vi "Lift_State_Machine.vi"() -> ()   [LabVIEW 2016]
doc: "The state machine for the Lift System.\nDrives the lift forward, then upward, then back, then down to its origin."
uses:
  <vilib>/myRIO/Instrument Drivers/Onboard IO/DIO/typedefs/DIO Reference.ctl
  <vilib>/myRIO/Common/Instrument Driver Framework/Utilities/typedefs/myRIO Generic Hardware Reference.ctl
  <vilib>/myRIO/Common/Instrument Driver Framework/Utilities/typedefs/Hardware Version Enum.ctl
  <vilib>/myRIO/Common/Instrument Driver Framework/Utilities/typedefs/myRIO v1.0 Reference.ctl
  <vilib>/myRIO/Common/Instrument Driver Framework/Utilities/typedefs/Generic FPGA Reference.ctl
  <vilib>/myRIO/Common/Instrument Driver Framework/myRIO v1.0/DIO/typedefs/DIO Channels List.ctl
  <vilib>/myRIO/Common/Instrument Driver Framework/myRIO v1.0/DIO/typedefs/DIO Channels Enum.ctl
  <vilib>/userdefined/High Color/nirio_resource_hc.ctl
  <vilib>/myRIO/Common/Instrument Driver Framework/Utilities/vis/Is FPGA Ref Available.vi
  <vilib>/myRIO/Common/Instrument Driver Framework/roboRIO v1.0/DIO/vis/roboRIO v1.0 Open DIO.vi
  <vilib>/myRIO/Instrument Drivers/Onboard IO/DIO/vis/Write.vi
  <vilib>/myRIO/Instrument Drivers/Onboard IO/DIO/vis/Read.vi
  <vilib>/myRIO/Common/Instrument Driver Framework/Utilities/vis/Validate Channels.vi
  <vilib>/myRIO/Common/Instrument Driver Framework/roboRIO v1.0/DIO/vis/roboRIO v1.0 Reserve DIO.vi
  <vilib>/myRIO/Common/Instrument Driver Framework/roboRIO v1.0/DIO/vis/roboRIO v1.0 Build MUX Configuration DIO.vi
  <vilib>/myRIO/Common/Instrument Driver Framework/roboRIO v1.0/Resource Manager/vis/roboRIO v1.0 Reserve Channel List.vi
  <vilib>/myRIO/Common/Instrument Driver Framework/roboRIO v1.0/Resource Manager/vis/roboRIO v1.0 Create Configuration List.vi
  <vilib>/myRIO/Common/Instrument Driver Framework/roboRIO v1.0/Resource Manager/vis/roboRIO v1.0 Reserve Channel.vi
  <vilib>/myRIO/Common/Instrument Driver Framework/roboRIO v1.0/Resource Manager/vis/roboRIO v1.0 Unreserve Channel.vi
  <vilib>/myRIO/Common/Instrument Driver Framework/roboRIO v1.0/Resource Manager/vis/roboRIO v1.0 Build Mutex Name.vi
  GlobalVI.vi
  <vilib>/Utility/VariantDataType/GetNumericInfo.vi
  <vilib>/Utility/error.llb/Error Cluster From Error Code.vi
  <vilib>/myRIO/Common/Instrument Driver Framework/roboRIO v1.0/roboRIO v1.0 Open.vi
  <vilib>/myRIO/Common/Instrument Driver Framework/Utilities/vis/IO Manager.vi
  <vilib>/myRIO/Common/Instrument Driver Framework/Utilities/vis/Configuration Manager.vi
  <vilib>/myRIO/Common/Instrument Driver Framework/roboRIO v1.0/Resource Manager/vis/roboRIO v1.0 Configure IO.vi
  <vilib>/myRIO/Common/Instrument Driver Framework/myRIO v1.0/myRIO v1.0 Close.vi
  <vilib>/myRIO/Common/Instrument Driver Framework/roboRIO v1.0/DIO/vis/roboRIO v1.0 Write DIO.vi
  <vilib>/myRIO/Common/Instrument Driver Framework/roboRIO v1.0/DIO/vis/roboRIO v1.0 Read DIO.vi
  <vilib>/myRIO/Express VI/Onboard IO/DO/DO Express VI.xnode
  <vilib>/myRIO/Instrument Drivers/Onboard IO/DIO/vis/myRIO DIO Open.xnode
  <vilib>/myRIO/Express VI/Onboard Devices/LED/LED Express VI.xnode
  <vilib>/myRIO/Express VI/Onboard IO/DI/DI Express VI.xnode
  <vilib>/myRIO/Instrument Drivers/Onboard IO/DIO/DIO.lvlib
panel:
  out "timeoutError":bool
  out "timeoutCounter":u32
  out "timerCount":u32
  out "liftState":i32
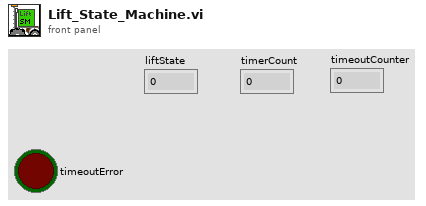
[diagram p1: front panel]
types:
  T1 = typedef "DIO.lvlib/DIO Reference.ctl" = cluster{"myRIO Reference":T2, "DIO Channels List":T6}
  T2 = typedef "myRIO Generic Hardware Reference.ctl" = cluster{"myRIO Model":T3, "myRIO Hardware Reference":T4}
  T3 = typedef "Hardware Version Enum.ctl" = enum16{"Unknown", "myRIO-1900", "myRIO-1950", "roboRIO", "NI ELVIS RIO CM"}
  T4 = typedef "myRIO v1.0 Reference.ctl" = cluster{"Generic FPGA Reference":T5, "Allow multiple opens":bool}
  T5 = typedef "Generic FPGA Reference.ctl" = refnum<k20>
  T6 = typedef "DIO Channels List.ctl" = T7[]
  T7 = typedef "DIO Channels Enum.ctl" = enum16{"Not Connected", "C/DIO0", "C/DIO1", "C/DIO2", "C/DIO3", "C/DIO4", "C/DIO5", "C/DIO6", "C/DIO7", "A/DIO0", "A/DIO1", "A/DIO2", "A/DIO3", "A/DIO4", "A/DIO5", "A/DIO6", "A/DIO7", "A/DIO8", "A/DIO9", "A/DIO10", "A/DIO11", "A/DIO12", "A/DIO13", "A/DIO14", "A/DIO15", "B/DIO0", "B/DIO1", "B/DIO2", "B/DIO3", "B/DIO4", "B/DIO5", "B/DIO6", "B/DIO7", "B/DIO8", "B/DIO9", "B/DIO10", "B/DIO11", "B/DIO12", "B/DIO13", "B/DIO14", "B/DIO15", "LED0", "LED1", "LED2", "LED3", "Button0", "DIO/DIO0", "DIO/DIO1", "DIO/DIO2", "DIO/DIO3", "DIO/DIO4", "DIO/DIO5", "DIO/DIO6", "DIO/DIO7", "DIO/DIO8", "DIO/DIO9", "SPI/CS0", "SPI/CS1", "SPI/CS2", "SPI/CS3", "LED RADIO (Green)", "LED RADIO (Red)", "LED COMM (Green)", "LED COMM (Red)", "LED MODE (Green)", "LED MODE (Red)"}
  T8 = typedef "nirio_resource_hc.ctl" = tag
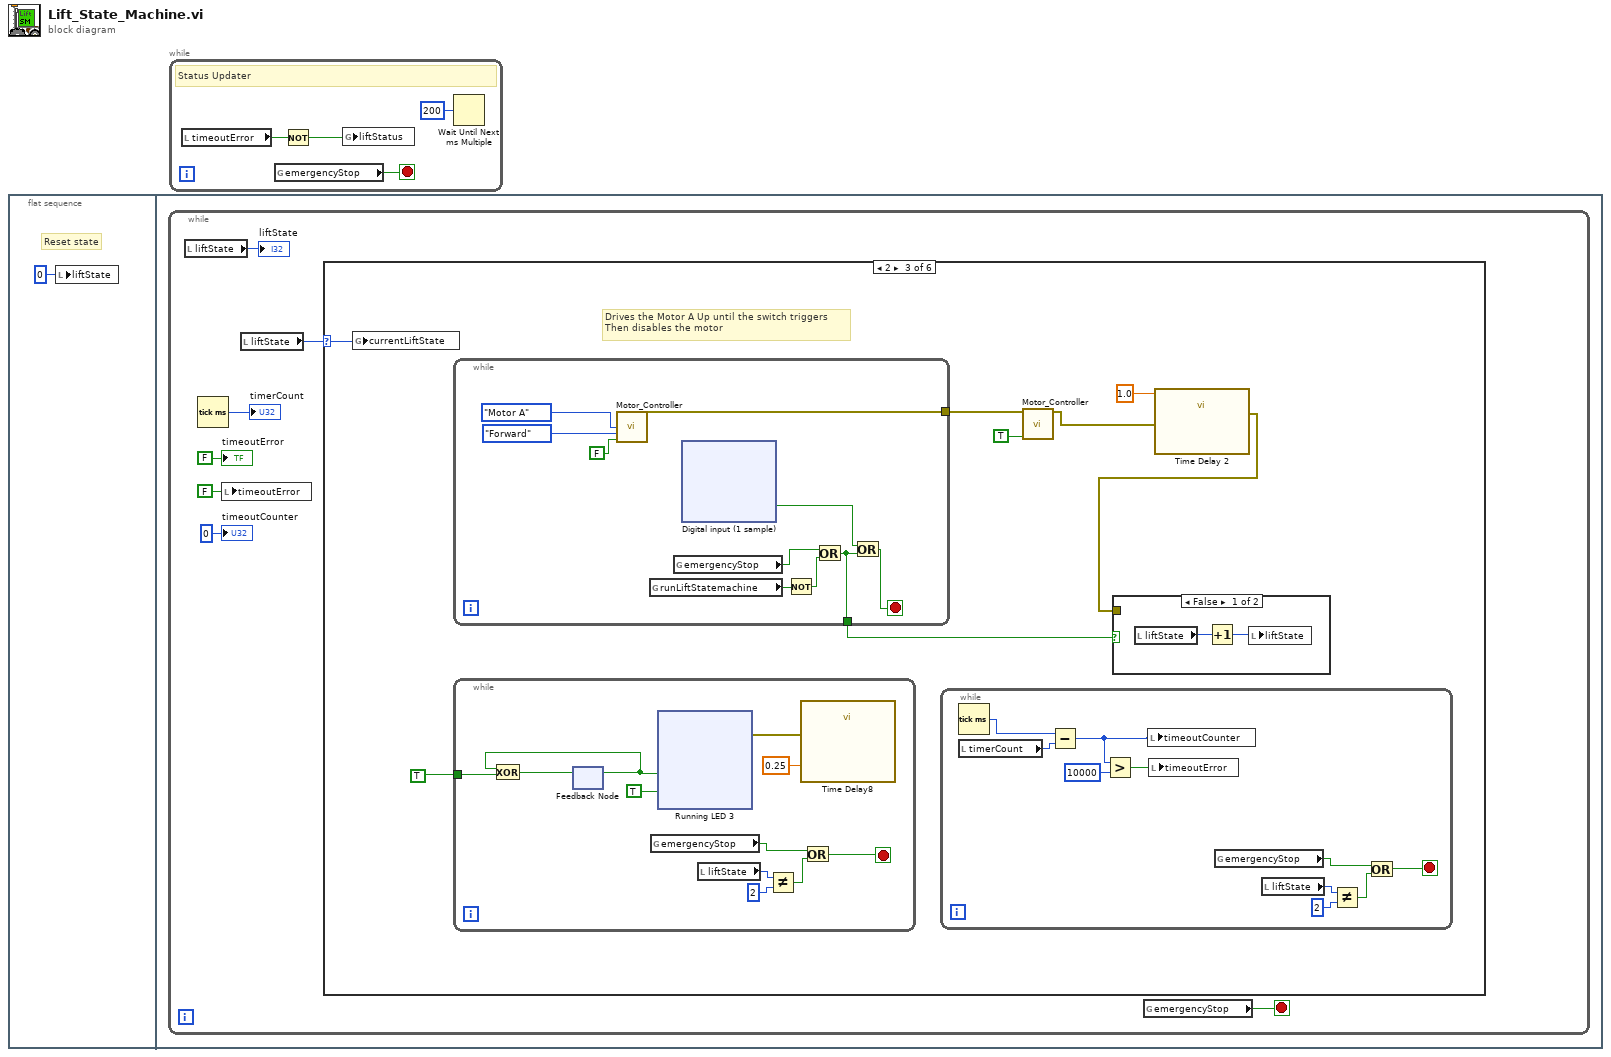
[diagram p0: block diagram]
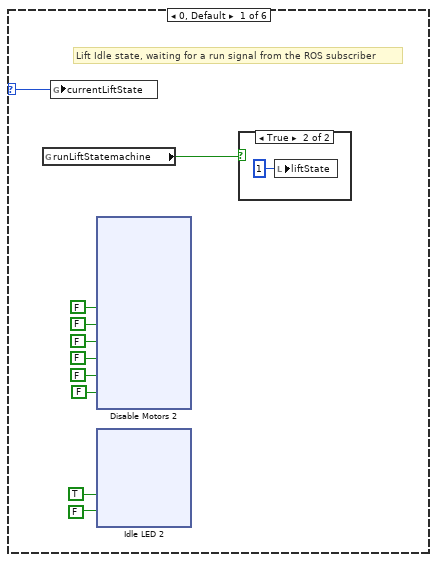
[diagram p2: hidden frame]
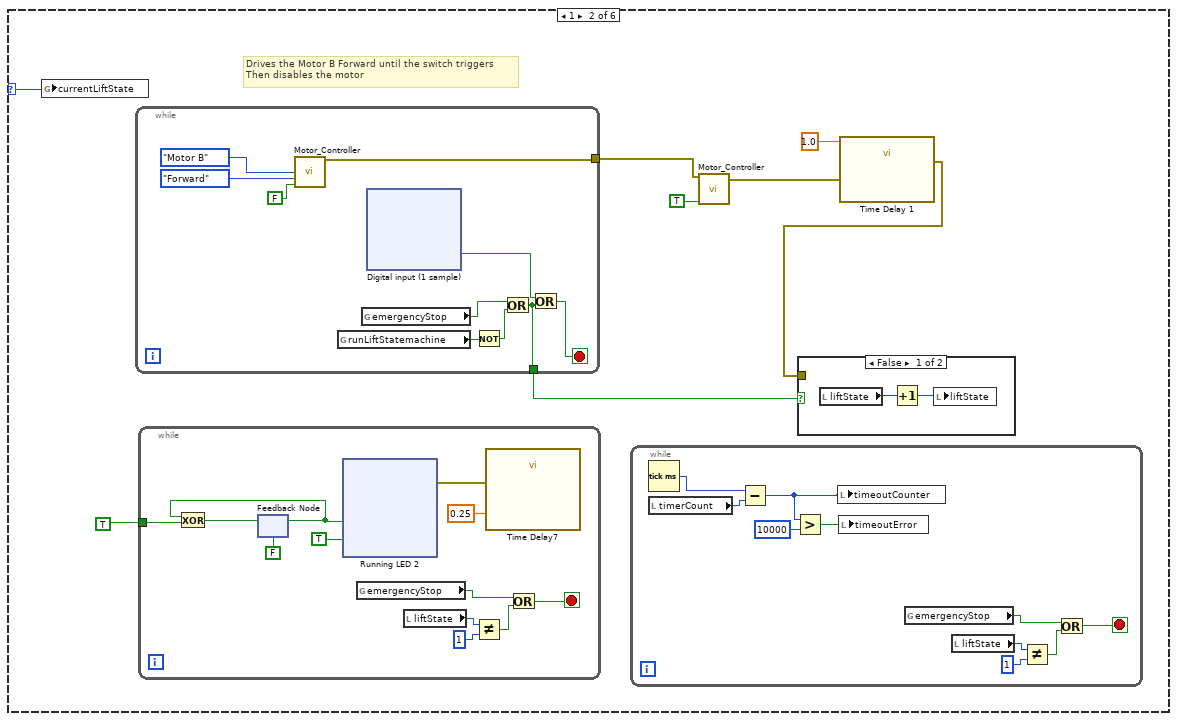
[diagram p4: hidden frame]
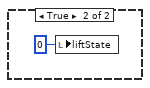
[diagram p5: hidden frame]
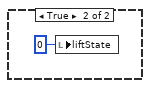
[diagram p6: hidden frame]
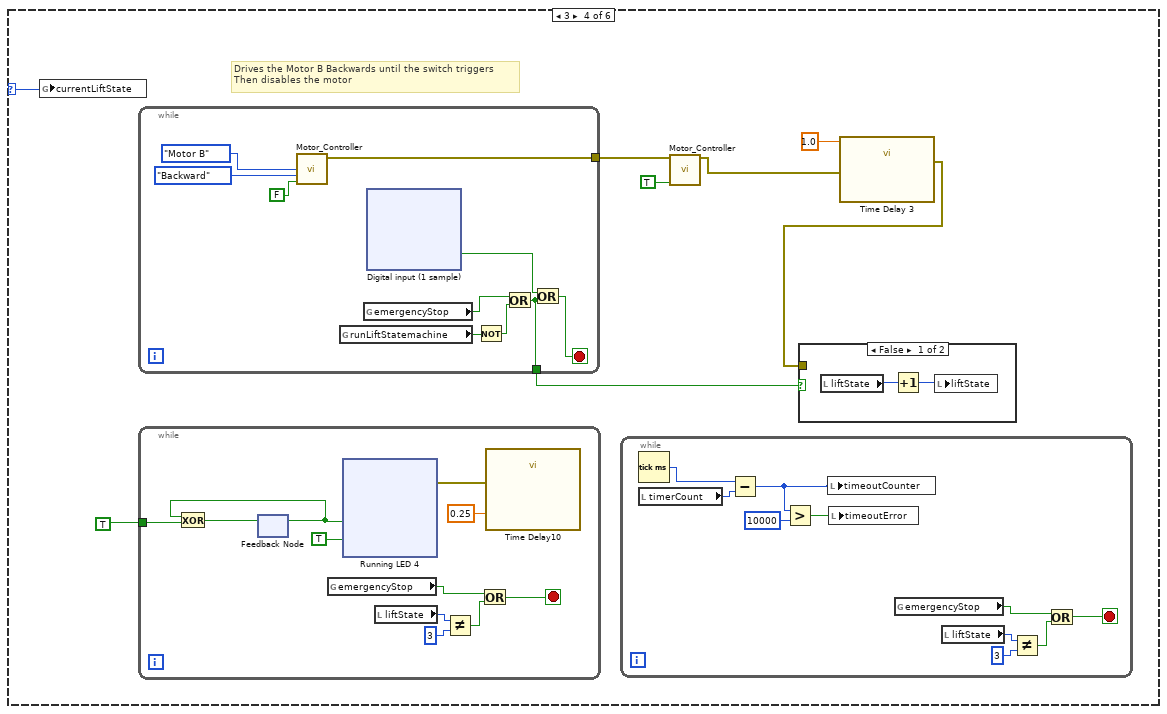
[diagram p7: hidden frame]
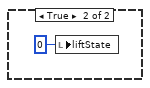
[diagram p8: hidden frame]
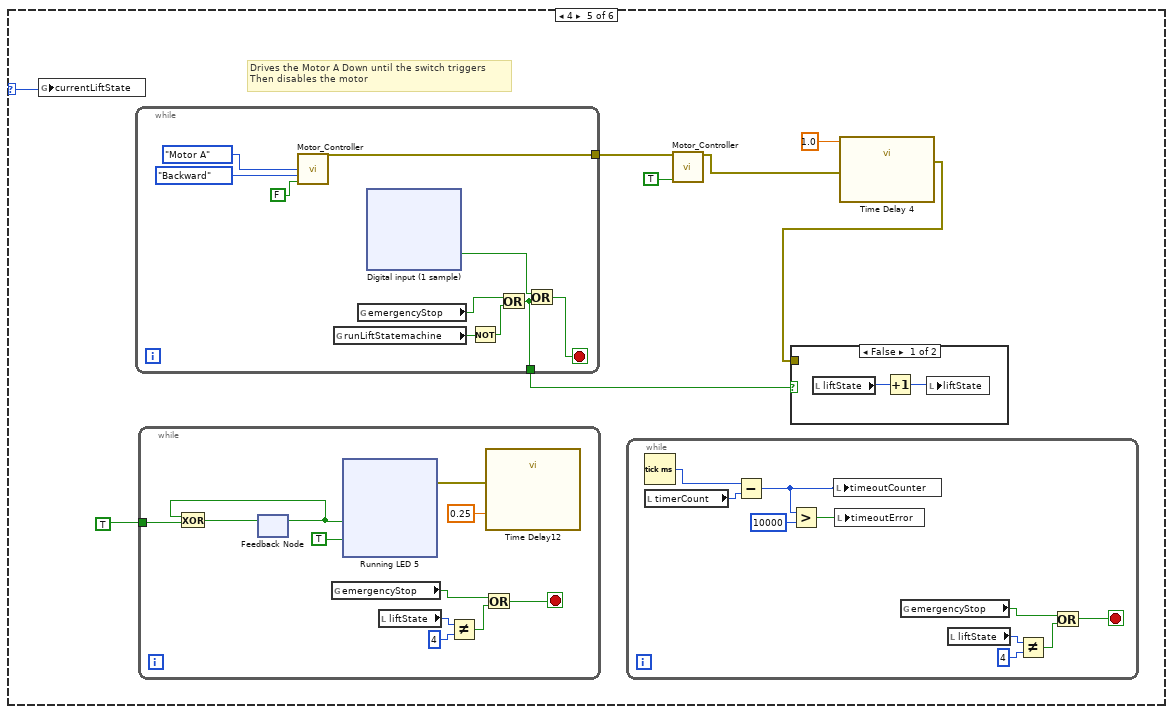
[diagram p9: hidden frame]
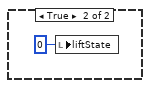
[diagram p10: hidden frame]
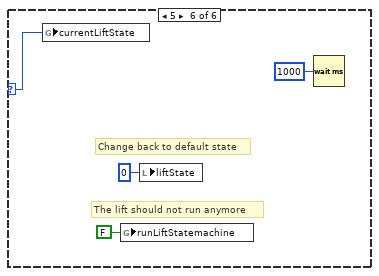
[diagram p11: hidden frame]
diagram:
  n1 = flat-sequence {
    frame #0 {
      # "Reset state"
      n2 = local write "liftState"(0 ("liftState")) -> ()
    }
    frame #1 {
      n3 = while {
        stop <- w8 stop-if-true
        n4 = local read "liftState"() -> (→"liftState":i32)
        n5 = Tick Count (ms)() -> (millisecond timer value=→"timerCount":u32)
        n6 = local write "timeoutError"(FALSE ("timeoutError")) -> ()
        n7 = local read "liftState"() -> (w6:i32)
        n8 = case shown="2" w6 {
          selector: w6 -> [w9 w96 w210 w323 w436 w551]
          frame 0, Default {
            # "Lift Idle state, waiting for a run signal from the ROS subscriber"
            n9 = global read "GlobalVI.vi" "runLiftStatemachine"() -> (w10:bool)
            n10 = global write "GlobalVI.vi" "currentLiftState"(w9) -> ()
            n11 = xnode "Disable Motors 2"("IN1 (B/DIO0 (Pin 11))"=FALSE, "IN2 (B/DIO1 (Pin 13))"=FALSE, "IN3 (B/DIO2 (Pin 15))"=FALSE, "IN4 (B/DIO3 (Pin 17))"=FALSE, "ENABLE A (B/DIO13 (Pin 26))"=FALSE, "ENABLE B (B/DIO8 (Pin 27))"=FALSE) -> ()  [unwired: 1 in, 1 out]
            n12 = xnode "Idle LED 2"("CommG"=TRUE, "CommR"=FALSE ("CommG")) -> ()  [unwired: 1 in, 1 out]
            n13 = case shown="True" w10 {
              frame False {
              }
              frame True {
                n14 = local write "liftState"(1 ("liftState")) -> ()
              }
            }
          }
          frame 1 {
            # "Drives the Motor B Forward until the switch triggers\nThen disables the motor"
            n15 = global write "GlobalVI.vi" "currentLiftState"(w96) -> ()
            n16 = while {
              tunnel: [w169] -> w97
              tunnel: [w170] -> w100
              stop <- w174 stop-if-true
              n17 = call "Motor_Controller.vi"("motorSelect"=enum16{"Motor A", "Motor B"}."Motor B", "direction"=enum16{"Forward", "Backward"}."Forward", "stopMotors"=FALSE) -> ("error out"=w169:errorcluster)  [unwired: 12 in]
              n18 = global read "GlobalVI.vi" "runLiftStatemachine"() -> (w173:bool)
              n19 = global read "GlobalVI.vi" "emergencyStop"() -> (w171:bool)
              n20 = xnode "Digital input (1 sample)"() -> ("B/DIO7 (Pin 25)"=w165:bool)  [unwired: 1 in, 1 out]
              n21 = Not(x=w173) -> (.not. x?=w172:bool)
              n22 = Or(x=w171, y=w172) -> (x .or. y?=w170:bool)
              n23 = Or(x=w165, y=w170) -> (x .or. y?=w174:bool)
            }
            n24 = while {
              tunnel: TRUE ("COMM (Red)") -> [w128]
              stop <- w118 stop-if-true
              n25 = feedback #1(FALSE) -> (w126:bool)
              n26 = Exclusive Or(1:w128, 2:w126) -> (0:w127:bool)
              n27 = feedback-in #1(w127) -> ()
              n28 = xnode "Running LED 2"("CommG"=w126, "CommR"=TRUE) -> ("error out"=w123:errorcluster)  [unwired: 1 in]
              n29 = global read "GlobalVI.vi" "emergencyStop"() -> (w119:bool)
              n30 = local read "liftState"() -> (w121:i32)
              n31 = Not Equal?(x=w121, y=1 ("liftState")) -> (x != y?=w120:bool)
              n32 = call "Time Delay7"("error in (no error)"=w123, "Delay Time (s)"=0.25) -> ()  [unwired: 9 in, 1 out]
              n33 = Or(x=w119, y=w120) -> (x .or. y?=w118:bool)
            }
            n34 = while {
              stop <- w107 stop-if-true
              n35 = Tick Count (ms)() -> (millisecond timer value=w113:u32)
              n36 = local read "timerCount"() -> (w112:u32)
              n37 = Subtract(x=w113, y=w112) -> (x-y=w104:u32)
              n38 = Greater?(x=w104, y=u32 10000) -> (0:w105:bool)
              n39 = local write "timeoutCounter"(w104) -> ()
              n40 = local write "timeoutError"(w105) -> ()
              n41 = global read "GlobalVI.vi" "emergencyStop"() -> (w111:bool)
              n42 = local read "liftState"() -> (w109:i32)
              n43 = Not Equal?(x=w109, y=1 ("liftState")) -> (x != y?=w110:bool)
              n44 = Or(x=w111, y=w110) -> (x .or. y?=w107:bool)
            }
            n45 = call "Motor_Controller.vi"("error in (no error)"=w97, "stopMotors"=TRUE) -> ("error out"=w98:errorcluster)  [unwired: 13 in]
            n46 = call "Time Delay 1"("error in (no error)"=w98, "Delay Time (s)"=1.0) -> ("error out"=w101:errorcluster)  [unwired: 9 in]
            n47 = case shown="False" w100 {
              tunnel: w101 -> [_ _]
              frame False {
                n48 = local read "liftState"() -> (w115:i32)
                n49 = Increment(x=w115) -> (x+1=w114:i32)
                n50 = local write "liftState"(w114) -> ()
              }
              frame True {
                n51 = local write "liftState"(0 ("liftState")) -> ()
              }
            }
          }
          frame 2 {
            # "Drives the Motor A Up until the switch triggers\nThen disables the motor"
            n52 = global write "GlobalVI.vi" "currentLiftState"(w210) -> ()
            n53 = while {
              tunnel: [w283] -> w214
              tunnel: [w280] -> w212
              stop <- w284 stop-if-true
              n54 = call "Motor_Controller.vi"("motorSelect"=enum16{"Motor A", "Motor B"}."Motor A", "direction"=enum16{"Forward", "Backward"}."Forward", "stopMotors"=FALSE) -> ("error out"=w280:errorcluster)  [unwired: 12 in]
              n55 = global read "GlobalVI.vi" "runLiftStatemachine"() -> (w287:bool)
              n56 = global read "GlobalVI.vi" "emergencyStop"() -> (w285:bool)
              n57 = xnode "Digital input (1 sample)"() -> ("B/DIO9 (Pin 29)"=w278:bool)  [unwired: 1 in, 1 out]
              n58 = Not(x=w287) -> (.not. x?=w286:bool)
              n59 = Or(x=w285, y=w286) -> (x .or. y?=w283:bool)
              n60 = Or(x=w278, y=w283) -> (x .or. y?=w284:bool)
            }
            n61 = while {
              tunnel: TRUE ("COMM (Red)") -> [w241]
              stop <- w231 stop-if-true
              n62 = feedback #2() -> (w239:bool)  [unwired: 1 in]
              n63 = Exclusive Or(1:w241, 2:w239) -> (0:w240:bool)
              n64 = feedback-in #2(w240) -> ()
              n65 = global read "GlobalVI.vi" "emergencyStop"() -> (w232:bool)
              n66 = xnode "Running LED 3"("CommG"=w239, "CommR"=TRUE) -> ("error out"=w236:errorcluster)  [unwired: 1 in]
              n67 = local read "liftState"() -> (w234:i32)
              n68 = Not Equal?(x=w234, y=2 ("liftState")) -> (x != y?=w233:bool)
              n69 = call "Time Delay8"("error in (no error)"=w236, "Delay Time (s)"=0.25) -> ()  [unwired: 9 in, 1 out]
              n70 = Or(x=w232, y=w233) -> (x .or. y?=w231:bool)
            }
            n71 = while {
              stop <- w221 stop-if-true
              n72 = Tick Count (ms)() -> (millisecond timer value=w227:u32)
              n73 = local read "timerCount"() -> (w226:u32)
              n74 = Subtract(x=w227, y=w226) -> (x-y=w218:u32)
              n75 = Greater?(x=w218, y=u32 10000) -> (0:w219:bool)
              n76 = local write "timeoutCounter"(w218) -> ()
              n77 = local write "timeoutError"(w219) -> ()
              n78 = global read "GlobalVI.vi" "emergencyStop"() -> (w225:bool)
              n79 = local read "liftState"() -> (w223:i32)
              n80 = Not Equal?(x=w223, y=2 ("liftState")) -> (x != y?=w224:bool)
              n81 = Or(x=w225, y=w224) -> (x .or. y?=w221:bool)
            }
            n82 = call "Motor_Controller.vi"("error in (no error)"=w212, "stopMotors"=TRUE) -> ("error out"=w211:errorcluster)  [unwired: 13 in]
            n83 = call "Time Delay 2"("error in (no error)"=w211, "Delay Time (s)"=1.0) -> ("error out"=w215:errorcluster)  [unwired: 9 in]
            n84 = case shown="False" w214 {
              tunnel: w215 -> [_ _]
              frame False {
                n85 = local read "liftState"() -> (w229:i32)
                n86 = Increment(x=w229) -> (x+1=w228:i32)
                n87 = local write "liftState"(w228) -> ()
              }
              frame True {
                n88 = local write "liftState"(0 ("liftState")) -> ()
              }
            }
          }
          frame 3 {
            # "Drives the Motor B Backwards until the switch triggers\nThen disables the motor"
            n89 = global write "GlobalVI.vi" "currentLiftState"(w323) -> ()
            n90 = while {
              tunnel: [w396] -> w327
              tunnel: [w393] -> w325
              stop <- w397 stop-if-true
              n91 = call "Motor_Controller.vi"("motorSelect"=enum16{"Motor A", "Motor B"}."Motor B", "direction"=enum16{"Forward", "Backward"}."Backward", "stopMotors"=FALSE) -> ("error out"=w393:errorcluster)  [unwired: 12 in]
              n92 = global read "GlobalVI.vi" "runLiftStatemachine"() -> (w400:bool)
              n93 = global read "GlobalVI.vi" "emergencyStop"() -> (w398:bool)
              n94 = xnode "Digital input (1 sample)"() -> ("B/DIO6 (Pin 23)"=w391:bool)  [unwired: 1 in, 1 out]
              n95 = Not(x=w400) -> (.not. x?=w399:bool)
              n96 = Or(x=w398, y=w399) -> (x .or. y?=w396:bool)
              n97 = Or(x=w391, y=w396) -> (x .or. y?=w397:bool)
            }
            n98 = while {
              tunnel: TRUE ("COMM (Red)") -> [w354]
              stop <- w344 stop-if-true
              n99 = feedback #3() -> (w352:bool)  [unwired: 1 in]
              n100 = Exclusive Or(1:w354, 2:w352) -> (0:w353:bool)
              n101 = feedback-in #3(w353) -> ()
              n102 = global read "GlobalVI.vi" "emergencyStop"() -> (w345:bool)
              n103 = xnode "Running LED 4"("CommG"=w352, "CommR"=TRUE) -> ("error out"=w349:errorcluster)  [unwired: 1 in]
              n104 = local read "liftState"() -> (w347:i32)
              n105 = Not Equal?(x=w347, y=3 ("liftState")) -> (x != y?=w346:bool)
              n106 = Or(x=w345, y=w346) -> (x .or. y?=w344:bool)
              n107 = call "Time Delay10"("error in (no error)"=w349, "Delay Time (s)"=0.25) -> ()  [unwired: 9 in, 1 out]
            }
            n108 = while {
              stop <- w334 stop-if-true
              n109 = Tick Count (ms)() -> (millisecond timer value=w340:u32)
              n110 = local read "timerCount"() -> (w339:u32)
              n111 = Subtract(x=w340, y=w339) -> (x-y=w331:u32)
              n112 = Greater?(x=w331, y=u32 10000) -> (0:w332:bool)
              n113 = local write "timeoutCounter"(w331) -> ()
              n114 = local write "timeoutError"(w332) -> ()
              n115 = global read "GlobalVI.vi" "emergencyStop"() -> (w338:bool)
              n116 = local read "liftState"() -> (w336:i32)
              n117 = Not Equal?(x=w336, y=3 ("liftState")) -> (x != y?=w337:bool)
              n118 = Or(x=w338, y=w337) -> (x .or. y?=w334:bool)
            }
            n119 = call "Motor_Controller.vi"("error in (no error)"=w325, "stopMotors"=TRUE) -> ("error out"=w324:errorcluster)  [unwired: 13 in]
            n120 = call "Time Delay 3"("error in (no error)"=w324, "Delay Time (s)"=1.0) -> ("error out"=w328:errorcluster)  [unwired: 9 in]
            n121 = case shown="False" w327 {
              tunnel: w328 -> [_ _]
              frame False {
                n122 = local read "liftState"() -> (w342:i32)
                n123 = Increment(x=w342) -> (x+1=w341:i32)
                n124 = local write "liftState"(w341) -> ()
              }
              frame True {
                n125 = local write "liftState"(0 ("liftState")) -> ()
              }
            }
          }
          frame 4 {
            # "Drives the Motor A Down until the switch triggers\nThen disables the motor"
            n126 = global write "GlobalVI.vi" "currentLiftState"(w436) -> ()
            n127 = while {
              tunnel: [w509] -> w441
              tunnel: [w506] -> w438
              stop <- w510 stop-if-true
              n128 = call "Motor_Controller.vi"("motorSelect"=enum16{"Motor A", "Motor B"}."Motor A", "direction"=enum16{"Forward", "Backward"}."Backward", "stopMotors"=FALSE) -> ("error out"=w506:errorcluster)  [unwired: 12 in]
              n129 = global read "GlobalVI.vi" "runLiftStatemachine"() -> (w513:bool)
              n130 = global read "GlobalVI.vi" "emergencyStop"() -> (w511:bool)
              n131 = xnode "Digital input (1 sample)"() -> ("B/DIO8 (Pin 27)"=w504:bool)  [unwired: 1 in, 1 out]
              n132 = Not(x=w513) -> (.not. x?=w512:bool)
              n133 = Or(x=w511, y=w512) -> (x .or. y?=w509:bool)
              n134 = Or(x=w504, y=w509) -> (x .or. y?=w510:bool)
            }
            n135 = while {
              tunnel: TRUE ("COMM (Red)") -> [w467]
              stop <- w457 stop-if-true
              n136 = feedback #4() -> (w465:bool)  [unwired: 1 in]
              n137 = Exclusive Or(1:w467, 2:w465) -> (0:w466:bool)
              n138 = feedback-in #4(w466) -> ()
              n139 = global read "GlobalVI.vi" "emergencyStop"() -> (w458:bool)
              n140 = xnode "Running LED 5"("CommG"=w465, "CommR"=TRUE) -> ("error out"=w462:errorcluster)  [unwired: 1 in]
              n141 = local read "liftState"() -> (w460:i32)
              n142 = Not Equal?(x=w460, y=4 ("liftState")) -> (x != y?=w459:bool)
              n143 = Or(x=w458, y=w459) -> (x .or. y?=w457:bool)
              n144 = call "Time Delay12"("error in (no error)"=w462, "Delay Time (s)"=0.25) -> ()  [unwired: 9 in, 1 out]
            }
            n145 = while {
              stop <- w447 stop-if-true
              n146 = Tick Count (ms)() -> (millisecond timer value=w453:u32)
              n147 = local read "timerCount"() -> (w452:u32)
              n148 = Subtract(x=w453, y=w452) -> (x-y=w444:u32)
              n149 = Greater?(x=w444, y=u32 10000) -> (0:w445:bool)
              n150 = local write "timeoutCounter"(w444) -> ()
              n151 = local write "timeoutError"(w445) -> ()
              n152 = global read "GlobalVI.vi" "emergencyStop"() -> (w451:bool)
              n153 = local read "liftState"() -> (w449:i32)
              n154 = Not Equal?(x=w449, y=4 ("liftState")) -> (x != y?=w450:bool)
              n155 = Or(x=w451, y=w450) -> (x .or. y?=w447:bool)
            }
            n156 = call "Motor_Controller.vi"("error in (no error)"=w438, "stopMotors"=TRUE) -> ("error out"=w437:errorcluster)  [unwired: 13 in]
            n157 = call "Time Delay 4"("error in (no error)"=w437, "Delay Time (s)"=1.0) -> ("error out"=w440:errorcluster)  [unwired: 9 in]
            n158 = case shown="False" w441 {
              tunnel: w440 -> [_ _]
              frame False {
                n159 = local read "liftState"() -> (w455:i32)
                n160 = Increment(x=w455) -> (x+1=w454:i32)
                n161 = local write "liftState"(w454) -> ()
              }
              frame True {
                n162 = local write "liftState"(0 ("liftState")) -> ()
              }
            }
          }
          frame 5 {
            # "The lift should not run anymore"
            # "Change back to default state"
            n163 = global write "GlobalVI.vi" "currentLiftState"(w551) -> ()
            n164 = global write "GlobalVI.vi" "runLiftStatemachine"(FALSE ("runLiftStatemachine")) -> ()
            n165 = local write "liftState"(0 ("liftState")) -> ()
            n166 = Wait (ms)(milliseconds to wait=u32 1000) -> ()  [unwired: 1 out]
          }
        }
        n167 = global read "GlobalVI.vi" "emergencyStop"() -> (w8:bool)
        "timeoutError" <- FALSE ("timeoutError")
        "timeoutCounter" <- u32 0 ("timeoutCounter")
      }
    }
  }
  n168 = while {
    stop <- w556 stop-if-true
    # "Status Updater"
    n169 = local read "timeoutError"() -> (w555:bool)
    n170 = global read "GlobalVI.vi" "emergencyStop"() -> (w556:bool)
    n171 = Not(x=w555) -> (.not. x?=w554:bool)
    n172 = global write "GlobalVI.vi" "liftStatus"(w554) -> ()
    n173 = Wait Until Next ms Multiple(millisecond multiple=u32 200) -> ()  [unwired: 1 out]
  }
